vi "EXA_Reference_Level_Y.vi"(0 "VISA resource name":refnum<visa-resource-name>, 5 "Mode":enum16{"Set", "Get"}(ring), 9 "Reference Level (dBm)":dbl, 11 "error in":errorcluster) -> (4 "VISA resource name":refnum<visa-resource-name>, 6 "Reference Level (dBm)":dbl, 15 "error out":errorcluster)   [LabVIEW 2016]
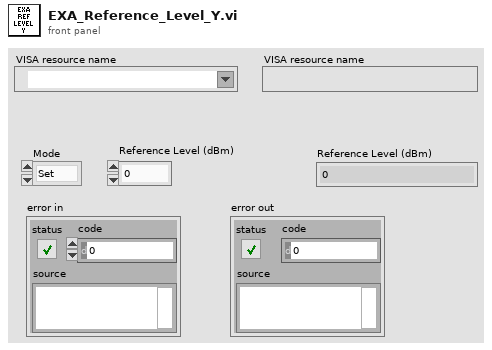
[diagram p1: front panel]
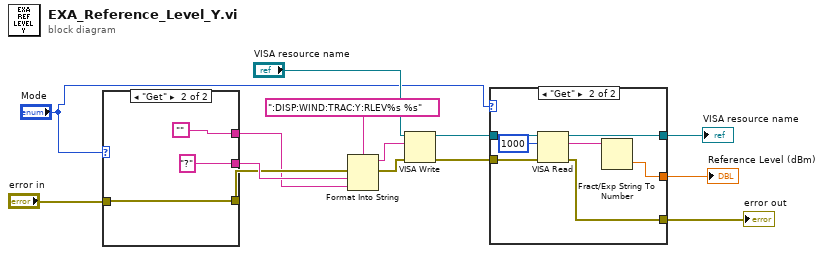
[diagram p0: block diagram]
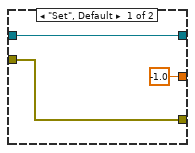
[diagram p2: hidden frame]
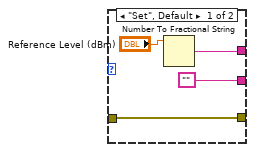
[diagram p3: hidden frame]
diagram:
  n1 = case shown="\"Get\"" "Mode" {
    tunnel: [w16 ""] -> w1
    tunnel: "error in" -> [w15 w20]
    tunnel: [w15 w20] -> w2
    tunnel: ["" "?"] -> w3
    frame "Set", Default {
      n2 = Number To Fractional String(number="Reference Level (dBm)") -> (F-format string=w16:string)  [unwired: 3 in]
    }
    frame "Get" {
    }
  }
  n3 = Format Into String(format string=":DISP:WIND:TRAC:Y:RLEV%s %s", error in=w2, w3, w1) -> (resulting string=w11:string, error out=w13:errorcluster)  [unwired: 1 in]
  n4 = VISA Write(VISA resource name="VISA resource name", write buffer=w11, error in (no error)=w13) -> (VISA resource name out=w7:refnum<visa-resource-name>, error out=w8:errorcluster)  [unwired: 1 out]
  n5 = case shown="\"Get\"" "Mode" {
    tunnel: w8 -> [w22 w31]
    tunnel: w7 -> [w24 w30]
    tunnel: [w24 w29] -> w4
    tunnel: [-1.0 w27] -> w6
    tunnel: [w22 w26] -> w5
    frame "Set", Default {
    }
    frame "Get" {
      n6 = VISA Read(VISA resource name=w30, byte count=u32 1000, error in (no error)=w31) -> (VISA resource name out=w29:refnum<visa-resource-name>, read buffer=w28:string, error out=w26:errorcluster)  [unwired: 1 out]
      n7 = Fract/Exp String To Number(string=w28) -> (number=w27:dbl)  [unwired: 3 in, 1 out]
    }
  }
  "error out" <- w5
  "VISA resource name" <- w4
  "Reference Level (dBm)" <- w6
